vi "LV FPGA Serial Read Write.vi"   [LabVIEW 2014]
uses:
  <vilib>/rvi/Emulation/niFpgaGetClockAttributes.vi
  <vilib>/rvi/Emulation/niFpgaSctlEmulationGetInTimedLoop.vi
  <vilib>/rvi/Emulation/niFpgaEmulationReportErrorSimple.vi
  Controls/Stop.vi
  <vilib>/rvi/eio/common/nirviEmuTemplateMethod_errors.vi
  <vilib>/rvi/Emulation/niFpgaCriticalErrorInLSC.vi
  <vilib>/rvi/Emulation/niFpgaEmulationIsFPGAContextNoSignature.vi
  <vilib>/rvi/errors/niFpgaSetErrorForExecOnDevCompSimple.vi
  <vilib>/rvi/eio/common/nirviEmuReportErrorAndStop.vi
  <vilib>/rvi/DataTransferAndStorage/Container/Common/niFpgaContainerGetUniqueNameForEmu.vi
  <vilib>/rvi/FIFO/Fifo_Resource/nirvififoEmulationSetSize.vi
  <vilib>/rvi/FIFO/Fifo_Resource/nirviFifoEmulationQueueMgr.vi
  <instcachedir>/0/nirviFifoEmulationQueueMgr_E5CAEC123FF24DC58D834DCA3CDAA9B5.lvgen/nirviFifoEmulationQueueMgr_E5CAEC123FF24DC58D834DCA3CDAA9B5_002.vi
  <vilib>/rvi/FIFO/Fifo_Resource/nirvififoEmulationDetermineInputValidOut.vi
  <vilib>/rvi/FIFO/Fifo_Resource/nirvififoEmulationCreateLock.vi
  <vilib>/rvi/Emulation/niFpgaProcessEmulError.vi
  <vilib>/rvi/FIFO/Fifo_Resource/nirvififoEmulationObtainLock.vi
  <vilib>/rvi/FIFO/Fifo_Resource/nirvififoEmulationReleaseLock.vi
  <vilib>/rvi/occurrence/nirviWaitOnOccurrenceBase.vi
  <vilib>/rvi/errors/nirviReportUnexpectedCaseInternalError.vi
  <vilib>/rvi/errors/nirviReportUnexpectedCaseInternalError (U32).vi
  <vilib>/eio/EIONode/EIONode.xnode
  <vilib>/rvi/DataTransferAndStorage/Container/XNode/niFpgaContainer.xnode
  <vilib>/rvi/FIFO/Fifo_Resource/nirvififoEmulationWrite.vi
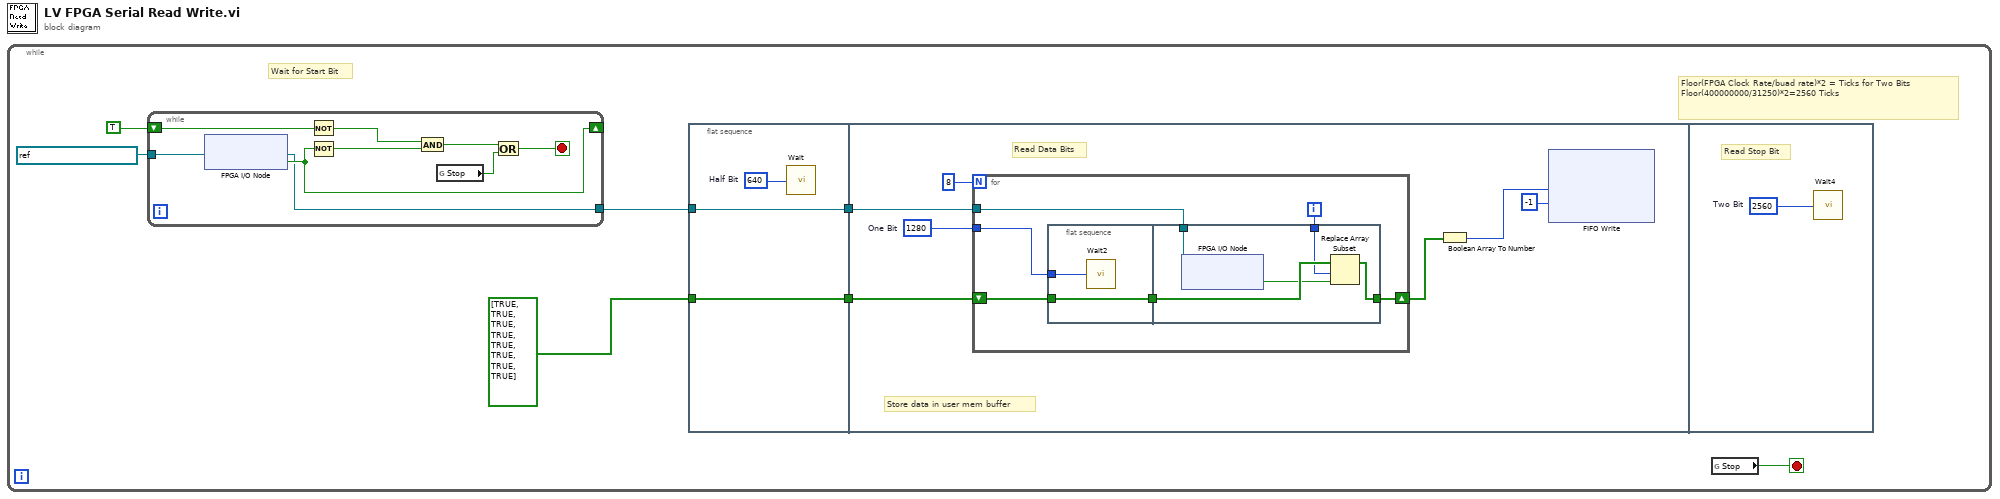
[diagram p0: block diagram]
diagram:
  n1 = while {
    stop <- w5 stop-if-true
    # "Floor(FPGA Clock Rate/buad rate)*2 = Ticks for Two Bits\nFloor(400000000/31250)*2=2560 Ticks"
    # "Wait for Start Bit"
    n2 = while {
      shift-right: [w33] -> _
      shift-left: TRUE -> [w40]
      tunnel: refnum<k21> "ConnectorA/DIO10" ("Receive") -> [w36]
      tunnel: [w32] -> w2
      stop <- w37 stop-if-true
      n3 = xnode "FPGA I/O Node"("FPGA I/O In"=w36) -> ("I/O Item"=w33:bool, "FPGA I/O Out"=w32:refnum<k21>)
      n4 = Not(x=w40) -> (.not. x?=w39:bool)
      n5 = Not(x=w33) -> (.not. x?=w34:bool)
      n6 = And(x=w39, y=w34) -> (x .and. y?=w38:bool)
      n7 = global read "Stop.vi" "Stop"() -> (w35:bool)
      n8 = Or(x=w38, y=w35) -> (x .or. y?=w37:bool)
    }
    n9 = flat-sequence {
      tunnel: [w10] -> w4
      tunnel: bool[] [TRUE, TRUE, TRUE, TRUE, TRUE, TRUE, TRUE, TRUE] -> [w10]
      tunnel: w2 -> [w8]
      tunnel: [w8] -> w1
      tunnel: w4 -> [w17]
      tunnel: w1 -> [w11]
      frame #0 {
        w9 = u32 640  # Half Bit
        n10 = call "Wait"("Count(Ticks)"=w9) -> ()  [unwired: 1 out]
      }
      frame #1 {
        w14 = u32 1280  # One Bit
        # "Store data in user mem buffer"
        # "Read Data Bits"
        n11 = for {
          N: 8 ("data bits (8)") -> [_]
          shift-right: [w20] -> w13
          shift-left: w17 -> [w23]
          tunnel: w14 -> [w21]
          tunnel: w11 -> [w19]
          i -> [w18]
          n12 = flat-sequence {
            tunnel: w23 -> [w25]
            tunnel: [w25] -> w22
            tunnel: w21 -> [w24]
            tunnel: w22 -> [w30]
            tunnel: [w29] -> w20
            tunnel: w19 -> [w28]
            tunnel: w18 -> [w27]
            frame #0 {
              n13 = call "Wait2"("Count(Ticks)"=w24) -> ()  [unwired: 1 out]
            }
            frame #1 {
              n14 = xnode "FPGA I/O Node"("FPGA I/O In"=w28) -> ("I/O Item"=w26:bool)  [unwired: 1 out]
              n15 = Replace Array Subset(array=w30, new element=w26, index=w27) -> (w29:bool[])
            }
          }
        }
        n16 = Boolean Array To Number(Boolean array=w13) -> (number=w12:u8)
        n17 = xnode ("FIFO Write")("Element"=w12, "Timeout"=-1) -> ()  [unwired: 1 in, 2 out]
      }
      frame #2 {
        w31 = u32 2560  # Two Bit
        # "Read Stop Bit"
        n18 = call "Wait4"("Count(Ticks)"=w31) -> ()  [unwired: 1 out]
      }
    }
    n19 = global read "Stop.vi" "Stop"() -> (w5:bool)
  }
